vi "Register.vi"(8 "error in (no error)":errorcluster, 11 "Test Executive Builder View in":refnum<class "Test Executive Builder View.lvclass">) -> (0 "error out":errorcluster, 3 "Test Executive Builder View out":refnum<class "Test Executive Builder View.lvclass">)   [LabVIEW 2017, in "Test Executive Builder View.lvclass"]
uses:
  Test Executive Builder View.lvclass
  C:/Program Files/National Instruments/LabVIEW 2017/vi.lib/gpm_packages/@cs/mva-core/Source/IObserver/IObserver/IObserver.lvclass
  <vilib>/gpm_packages/@cs/mva-core/Source/SubscriptionPolicy/BasicSubscription/BasicSubscription.lvclass
  C:/Program Files/National Instruments/LabVIEW 2017/vi.lib/gpm_packages/@cs/mva-core/Source/IMediator/ISubscriptionPolicy/ISubscriptionPolicy.lvclass
  Test Executive Builder View Messages/Draw Tree Msg/Draw Tree Msg.lvclass
  C:/Program Files/National Instruments/LabVIEW 2017/vi.lib/gpm_packages/@cs/transport/Source/Concrete/ActorMessageTransport/Notification Msg/Notification Msg.lvclass
  <vilib>/gpm_packages/@cs/mva-core/Source/SubscriptionPolicy/BasicSubscription/BasicSubscription.lvclass/BasicSubscription.ctl
  <vilib>/ActorFramework/Actor/Actor.lvclass/Actor.ctl
  <vilib>/ActorFramework/Message Enqueuer/Message Enqueuer.lvclass/Message Enqueuer.ctl
  <vilib>/gpm_packages/@cs/transport/Source/Concrete/ActorMessageTransport/ActorMessageTransport.lvclass/ActorMessageTransport.ctl
  <vilib>/gpm_packages/@cs/mva-core/Source/IMediator/SubscriptionRequest/SubscriptionRequest.lvclass/SubscriptionRequest.ctl
  <vilib>/gpm_packages/@cs/mva-core/Source/IObserver/IObserver Messages/Subscribe Msg/Subscribe Msg.lvclass/Subscribe Msg.ctl
  <vilib>/gpm_packages/@cs/mva-core/Source/IMediator/SubscriptionRequest/Pack Subscription Request.vi
  <vilib>/gpm_packages/@cs/mva-core/Source/IObserver/IObserver Messages/Subscribe Msg/Send Subscribe.vi
  <vilib>/ActorFramework/Actor/Read Self Enqueuer.vi
  <vilib>/gpm_packages/@cs/transport/Source/Concrete/ActorMessageTransport/Construct Actor Message Transport.vi
  <vilib>/ActorFramework/Message Enqueuer/Enqueue.vi
  <vilib>/ActorFramework/Message Enqueuer/Init from Existing Queue.vi
  <vilib>/ActorFramework/Message Enqueuer/Equals Not A Refnum.vi
  <vilib>/gpm_packages/@cs/mva-core/Source/IObserver/IObserver/IObserver.lvclass
  C:/Program Files/National Instruments/LabVIEW 2017/vi.lib/ActorFramework/Actor/Actor.lvclass
  <vilib>/gpm_packages/@cs/transport/Source/Concrete/ActorMessageTransport/ActorMessageTransport.lvclass
  C:/Program Files/National Instruments/LabVIEW 2017/vi.lib/gpm_packages/@cs/transport/Source/ITransport/ITransport.lvclass
  <vilib>/gpm_packages/@cs/mva-core/Source/IObserver/IObserver Messages/Subscribe Msg/Subscribe Msg.lvclass
  C:/Program Files/National Instruments/LabVIEW 2017/vi.lib/ActorFramework/Message/Message.lvclass
  <vilib>/Utility/error.llb/Error Cluster From Error Code.vi
  <vilib>/gpm_packages/@cs/mva-core/Source/IMediator/ISubscriptionPolicy/Open Subscription Policy.vi
  <vilib>/ActorFramework/Message Priority Queue/Priority Enqueue.vi
  <vilib>/ActorFramework/Message Enqueuer/Message Enqueuer.lvclass
  <vilib>/gpm_packages/@cs/mva-core/Source/IMediator/SubscriptionRequest/SubscriptionRequest.lvclass
  <vilib>/gpm_packages/@cs/transport/Source/Concrete/ActorMessageTransport/Notification Msg/Notification Msg.lvclass
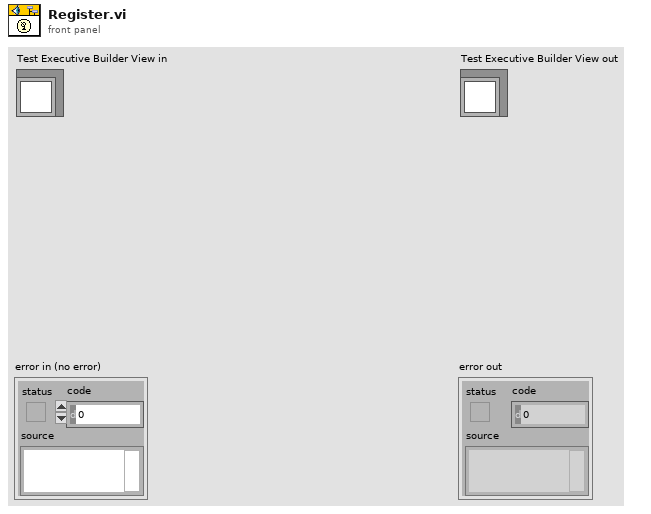
[diagram p1: front panel]
types:
  T1 = cluster{"Left Cell String":string, "Child Text":string[], "Child Tag":string, "Item Indent":i32, "Child Only?":bool, "Glyph Index":i32}[]
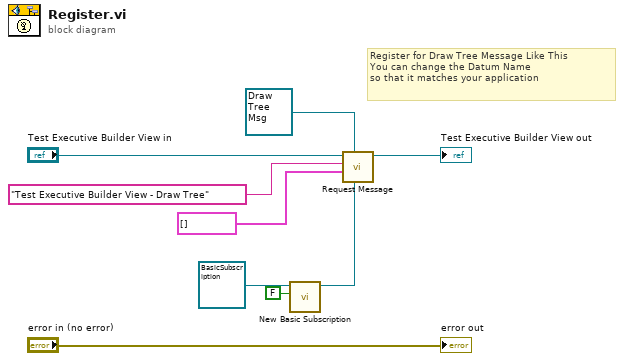
[diagram p0: block diagram]
diagram:
  # "Register for Draw Tree Message Like This\nYou can change the Datum Name \nso that it matches your application"
  n1 = call <vilib>:"New Basic Subscription.vi"("Ignore Past Updates? (F)"=FALSE, "BasicSubscription In"=refnum<class "BasicSubscription.lvclass"> refnum ("SubscriptionPolicy.lvlib:BasicSubscription.lvclass")) -> ("BasicSubscription Out"=w6:refnum<class "BasicSubscription.lvclass">)  [unwired: 9 in]
  n2 = call <vilib>:"Request Message.vi"("Configured SubscriptionPolicy"=w6, "Desired Notification Msg"=refnum<class "Draw Tree Msg.lvclass"> refnum ("Test Executive Builder View.lvlib:Draw Tree Msg.lvclass"), "Data Type"=T1 [] ("Tree Data"), "Datum Name"="Test Executive Builder View - Draw Tree", "IObserver in"="Test Executive Builder View in") -> ("IObserver out"=→"Test Executive Builder View out":refnum<class "Test Executive Builder View.lvclass">)  [unwired: 4 in, 2 out]
  "error out" <- "error in (no error)"
